vi "Initialize.vi"(8 "error in (no error)":errorcluster, 10 "Main VI":refnum<vi>, 11 "Numeric Data Type in":refnum<class "Numeric Data Type.lvclass">) -> (0 "error out":errorcluster, 3 "Numeric Data Type out":refnum<class "Numeric Data Type.lvclass">)   [LabVIEW 2018, in "Numeric Data Type.lvclass"]
uses:
  Numeric Data Type.lvclass
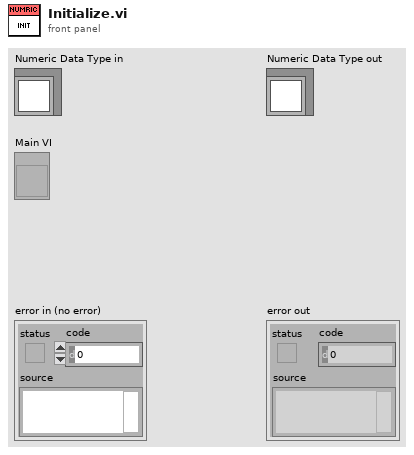
[diagram p1: front panel]
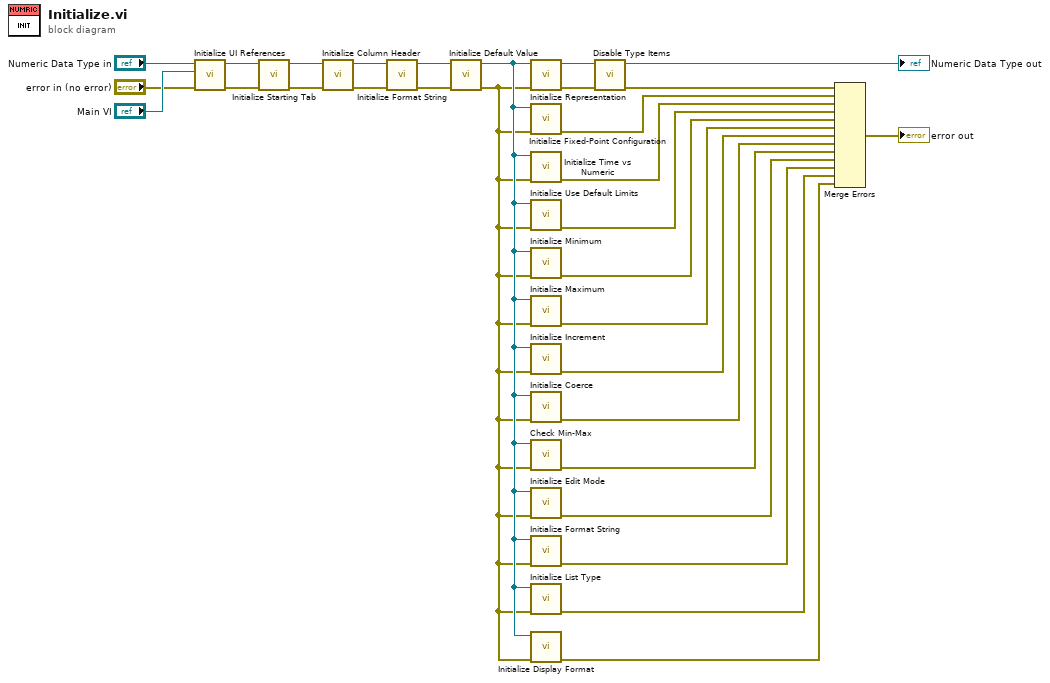
[diagram p0: block diagram]
diagram:
  n1 = call "Initialize UI References.vi"("error in (no error)"="error in (no error)", "VI Refnum"="Main VI", "Numeric Data Type in"="Numeric Data Type in") -> ("error out"=w6:errorcluster, "Numeric Data Type out"=w8:refnum<class "Numeric Data Type.lvclass">)  [unwired: 7 in]
  n2 = call "Initialize Starting Tab.vi"("error in (no error)"=w6, "Numeric Data Type in"=w8) -> ("error out"=w5:errorcluster, "Numeric Data Type out"=w7:refnum<class "Numeric Data Type.lvclass">)  [unwired: 8 in]
  n3 = call "Initialize Column Header.vi"("error in (no error)"=w5, "Numeric Data Type in"=w7) -> ("error out"=w9:errorcluster, "Numeric Data Type out"=w10:refnum<class "Numeric Data Type.lvclass">)  [unwired: 8 in]
  n4 = call "Initialize Format String.vi"("error in (no error)"=w9, "Numeric Data Type in"=w10) -> ("error out"=w2:errorcluster, "Numeric Data Type (dup)"=w4:refnum<class "Numeric Data Type.lvclass">)  [unwired: 8 in]
  n5 = call "Initialize Default Value.vi"("error in (no error)"=w2, "Numeric Data Type in"=w4) -> ("error out"=w1:errorcluster, "Numeric Data Type (dup)"=w3:refnum<class "Numeric Data Type.lvclass">)  [unwired: 8 in]
  n6 = call "Initialize Representation.vi"("error in (no error)"=w1, "Numeric Data Type in"=w3) -> ("error out"=w13:errorcluster, "Numeric Data Type (dup)"=w15:refnum<class "Numeric Data Type.lvclass">)  [unwired: 8 in]
  n7 = call "Initialize Fixed-Point Configuration.vi"("error in (no error)"=w1, "Numeric Data Type in"=w3) -> ("error out"=w26:errorcluster)  [unwired: 8 in, 1 out]
  n8 = call "Initialize Time vs Numeric.vi"("error in (no error)"=w1, "Numeric Data Type in"=w3) -> ("error out"=w25:errorcluster)  [unwired: 8 in, 1 out]
  n9 = call "Initialize Use Default Limits.vi"("error in (no error)"=w1, "Numeric Data Type in"=w3) -> ("error out"=w24:errorcluster)  [unwired: 8 in, 1 out]
  n10 = call "Initialize Minimum.vi"("error in (no error)"=w1, "Numeric Data Type in"=w3) -> ("error out"=w23:errorcluster)  [unwired: 8 in, 1 out]
  n11 = call "Initialize Maximum.vi"("error in (no error)"=w1, "Numeric Data Type in"=w3) -> ("error out"=w22:errorcluster)  [unwired: 8 in, 1 out]
  n12 = call "Initialize Increment.vi"("error in (no error)"=w1, "Numeric Data Type in"=w3) -> ("error out"=w21:errorcluster)  [unwired: 8 in, 1 out]
  n13 = call "Initialize Coerce.vi"("error in (no error)"=w1, "Numeric Data Type in"=w3) -> ("error out"=w20:errorcluster)  [unwired: 8 in, 1 out]
  n14 = call "Check Min-Max.vi"("error in (no error)"=w1, "Numeric Data Type in"=w3) -> ("error out"=w19:errorcluster)  [unwired: 8 in, 1 out]
  n15 = call "Initialize Edit Mode.vi"("error in (no error)"=w1, "Numeric Data Type in"=w3) -> ("error out"=w18:errorcluster)  [unwired: 8 in, 1 out]
  n16 = call "Initialize Format String.vi"("error in (no error)"=w1, "Numeric Data Type in"=w3) -> ("error out"=w11:errorcluster)  [unwired: 8 in, 1 out]
  n17 = call "Initialize List Type.vi"("error in (no error)"=w1, "Numeric Data Type in"=w3) -> ("error out"=w17:errorcluster)  [unwired: 8 in, 1 out]
  n18 = call "Initialize Display Format.vi"("error in (no error)"=w1, "Numeric Data Type in"=w3) -> ("error out"=w16:errorcluster)  [unwired: 8 in, 1 out]
  n19 = call "Disable Type Items.vi"("error in (no error)"=w13, "Numeric Data Type in"=w15) -> ("error out"=w12:errorcluster, "Numeric Data Type out"=→"Numeric Data Type out":refnum<class "Numeric Data Type.lvclass">)  [unwired: 8 in]
  n20 = Merge Errors(w12, w26, w25, w24, w23, w22, w21, w20, w19, w18, w11, w17, w16) -> (→"error out":errorcluster)
